vi "Enqueue Blocks.vi"(10 "data":u8[](array[numeric]) format="%.0x", 11 "Blocks queue":refnum<queue>) -> ()   [LabVIEW 2013, in "MD5.lvlib" / "MD5.lvclass"]
uses:
  MD5.lvclass
  Data-vector.ctl
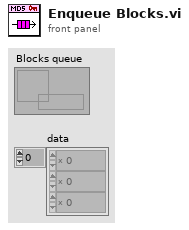
[diagram p1: front panel]
types:
  T1 = typedef "MD5.lvlib/MD5.lvclass/Data-vector.ctl" = cluster{"Data[ ]":u8[], "end":bool}
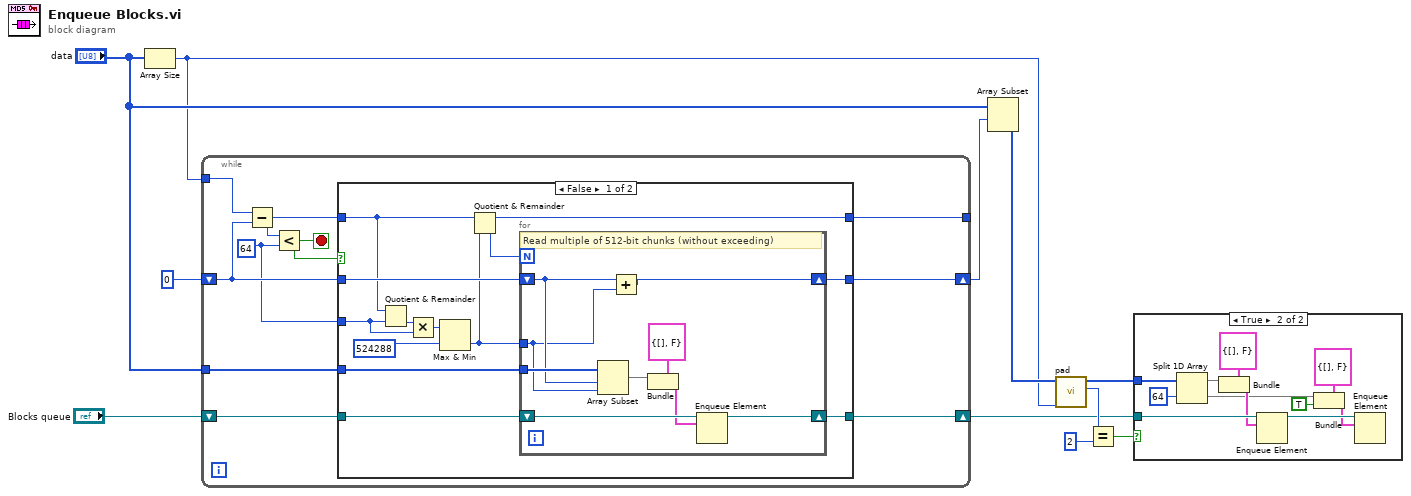
[diagram p0: block diagram]
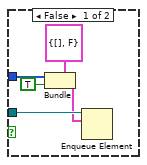
[diagram p3: hidden frame]
diagram:
  n1 = Array Size(array="data") -> (size(s)=w1:i32)
  n2 = while {
    shift-right: [w17] -> w4
    shift-left: 0 ("offset") -> [w19]
    tunnel: w1 -> [w15]
    tunnel: [w18] -> _
    tunnel: "data" -> [w16]
    shift-right: [w20] -> w5
    shift-left: "Blocks queue" -> [w21]
    stop <- w12 stop-if-true
    w13 = 64 ("y")
    n3 = Subtract(x=w15, y=w19) -> (x-y=w14:i32)
    n4 = Less?(x=w14, y=w13) -> (x < y?=w12:bool)
    n5 = case shown="False" w12 {
      tunnel: w21 -> [w34 w44]
      tunnel: [w33 w44] -> w20
      tunnel: w19 -> [w32 w45]
      tunnel: [w26 _] -> w18
      tunnel: [w25 w45] -> w17
      tunnel: w16 -> [w24 _]
      tunnel: w14 -> [w23 _]
      tunnel: w13 -> [w22 _]
      frame False {
        n6 = Quotient & Remainder(x=w23, y=w22) -> (floor(x/y)=w31:i32)  [unwired: 1 out]
        n7 = Multiply(x=w31, y=w22) -> (x*y=w30:i32)
        n8 = Max & Min(x=w30, y=524288) -> (min(x,y)=w27:i32)  [unwired: 1 out]
        n9 = Quotient & Remainder(x=w23, y=w27) -> (x-y*floor(x/y)=w26:i32, floor(x/y)=w28:i32)
        n10 = for {
          N: w28 -> [_]
          shift-right: [w42] -> w33
          shift-left: w34 -> [w43]
          shift-right: [w35] -> w25
          shift-left: w32 -> [w37]
          tunnel: w27 -> [w36]
          tunnel: w24 -> [w39]
          # "Read multiple of 512-bit chunks (without exceeding)"
          n11 = Array Subset(array=w39, index=w37, length=w36) -> (w38:u8[])
          n12 = Add(x=w37, y=w36) -> (x+y=w35:i32)
          n13 = Bundle(cluster=T1 {"Data[ ]"=[], "end"=FALSE}, "Data[ ]"=w38) -> (w40:T1)  [unwired: 1 in]
          n14 = Enqueue Element(queue=w43, element=w40) -> (queue out=w42:refnum<queue>)  [unwired: 2 in, 2 out]
        }
      }
      frame True {
      }
    }
  }
  n15 = Array Subset(array="data", index=w4) -> (w2:u8[])  [unwired: 1 in]
  n16 = call "pad.vi"("data length"=w1, "Last Block"=w2) -> ("blocks"=w9:i32, "Padding"=w8:u8[])  [unwired: 8 in]
  n17 = Equal?(x=w9, y=2) -> (x = y?=w11:bool)
  n18 = case shown="True" w11 {
    tunnel: w5 -> [w47 w61]
    tunnel: w8 -> [w49 w60]
    frame False {
      n19 = Bundle(cluster=T1 {"Data[ ]"=[], "end"=FALSE}, "Data[ ]"=w49, "end"=TRUE) -> (w46:T1)
      n20 = Enqueue Element(queue=w47, element=w46) -> ()  [unwired: 2 in, 3 out]
    }
    frame True {
      n21 = Split 1D Array(array=w60, index=64) -> (first subarray=w56:u8[], second subarray=w53:u8[])
      n22 = Bundle(cluster=T1 {"Data[ ]"=[], "end"=FALSE}, "Data[ ]"=w56) -> (w58:T1)  [unwired: 1 in]
      n23 = Enqueue Element(queue=w61, element=w58) -> (queue out=w55:refnum<queue>)  [unwired: 2 in, 2 out]
      n24 = Bundle(cluster=T1 {"Data[ ]"=[], "end"=FALSE}, "Data[ ]"=w53, "end"=TRUE) -> (w51:T1)
      n25 = Enqueue Element(queue=w55, element=w51) -> ()  [unwired: 2 in, 3 out]
    }
  }
